vi "Load Complete.vi"(8 "error in (no error)":errorcluster, 11 "Application Controller in":refnum<class "Application Controller.lvclass">) -> (0 "error out":errorcluster, 3 "Application Controller out":refnum<class "Application Controller.lvclass">)   [LabVIEW 2016, in "Application Controller.lvclass"]
uses:
  Application Controller.lvclass
  C:/Program Files/National Instruments/LabVIEW 2016/vi.lib/ActorFramework/Actor/Actor.lvclass
  <vilib>/ActorFramework/Actor/Actor.lvclass/Actor.ctl
  <vilib>/ActorFramework/Message Enqueuer/Message Enqueuer.lvclass/Message Enqueuer.ctl
  Application Controller.lvclass/Application Controller.ctl
  Read Launch Notifier.vi
  <vilib>/ActorFramework/Message Enqueuer/Init from Existing Queue.vi
  <vilib>/ActorFramework/Message Enqueuer/Enqueue.vi
  Template Module Messages/Open Front Panel Msg/Open Front Panel Msg.lvclass
  C:/Program Files/National Instruments/LabVIEW 2016/vi.lib/ActorFramework/Message/Message.lvclass
  <vilib>/ActorFramework/Message Priority Queue/Priority Enqueue.vi
  <vilib>/ActorFramework/Message Enqueuer/Message Enqueuer.lvclass
  <vilib>/ActorFramework/Actor/Actor.lvclass
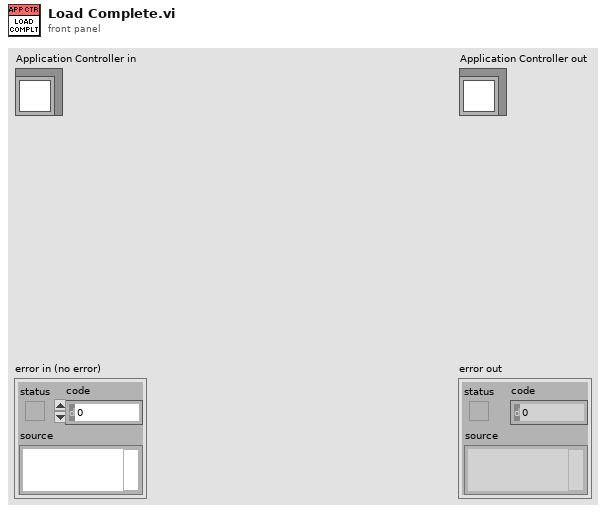
[diagram p1: front panel]
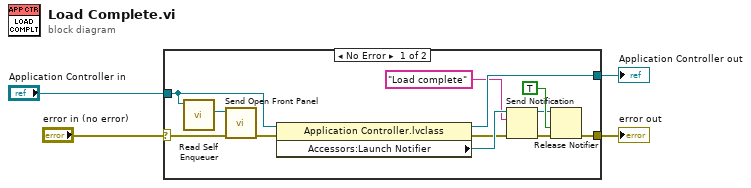
[diagram p0: block diagram]
diagram:
  n1 = case shown="No Error" "error in (no error)" {
    selector: "error in (no error)" -> [w8 w18]
    tunnel: [w6 w18] -> w3
    tunnel: [w13 w17] -> w1
    tunnel: "Application Controller in" -> [w10 w17]
    frame No Error {
      n2 = call <vilib>:"Read Self Enqueuer.vi"("Actor"=w10) -> ("Self Enqueuer"=w9:refnum<class "Message Enqueuer.lvclass">)  [unwired: 10 in]
      n3 = call "Send Open Front Panel.vi"("error in (no error)"=w8, "Message Enqueuer"=w9) -> ("error out"=w5:errorcluster)  [unwired: 8 in, 1 out]
      n4 = property class="Application Controller.lvclass"(reference=w10, error in=w5) -> (reference out=w13:refnum<class "Application Controller.lvclass">, error out=w7:errorcluster, "Accessors:Launch Notifier"=w12:refnum<notifier>)
      n5 = Send Notification(notification="Load complete" ("Message"), notifier=w12, error in (no error)=w7) -> (notifier out=w14:refnum<notifier>, error out=w15:errorcluster)
      n6 = Release Notifier(notifier=w14, force destroy? (F)=TRUE ("Kill notifier"), error in (no error)=w15) -> (error out=w6:errorcluster)  [unwired: 2 out]
    }
    frame Error {
    }
  }
  "error out" <- w3
  "Application Controller out" <- w1
